vi "Zähler_konfigurieren_FGV.vi"(0 "Band/Station Index":T4, 1 "Modus":T3(ring), 3 "Konfiguration":T2, 4 "Zähler":enum16{"Zähler 1", "Zähler 2", "Zähler 3"}(ring)) -> (6 "Zählerkonfig.":T1(array[cluster]), 7 "Werte verändert":bool)   [LabVIEW 2013, in "cRIO_FPGA_COMMUNICATION.lvlib"]
uses:
  TYPES/TYPE Station Index.ctl
  cRIO_FPGA_COMMUNICATION.lvlib
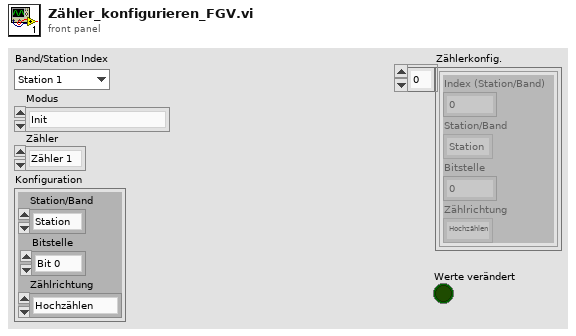
[diagram p1: front panel]
types:
  T1 = cluster{"Index (Station/Band)":u8, "Station/Band":enum16{"Station", "Band"}, "Bitstelle":u8, "Zählrichtung":enum16{"Hochzählen", "Runterzählen"}}[]
  T2 = typedef "TYPE Zählerkonfiguration.ctl" = cluster{"Station/Band":enum16{"Station", "Band"}, "Bitstelle":enum16{"Bit 0", "Bit 1", "Bit 2", "Bit 3", "Bit 4", "Bit 5", "Bit 6", "Bit 7"}, "Zählrichtung":enum16{"Hochzählen", "Runterzählen"}}
  T3 = enum16{"Init", "Zählerkonfig. setzen", "lese Zählerkonfig."}
  T4 = typedef "cRIO_FPGA_COMMUNICATION.lvlib/TYPE Station Index.ctl" = enum16{"Station 1", "Station 2", "Station 3", "Station 4", "Station 5", "Station 6", "Station 7", "Station 8", "Station 9", "Station 10", "Station 11", "Station 12", "Station 13", "Station 14", "Station 15", "Station 16", "Station 17", "Station 18", "Station 19", "Station 20"}
  T5 = cluster{"Index (Station/Band)":u8, "Station/Band":enum16{"Station", "Band"}, "Bitstelle":u8, "Zählrichtung":enum16{"Hochzählen", "Runterzählen"}}
  T6 = enum16{"Bit 0", "Bit 1", "Bit 2", "Bit 3", "Bit 4", "Bit 5", "Bit 6", "Bit 7"}
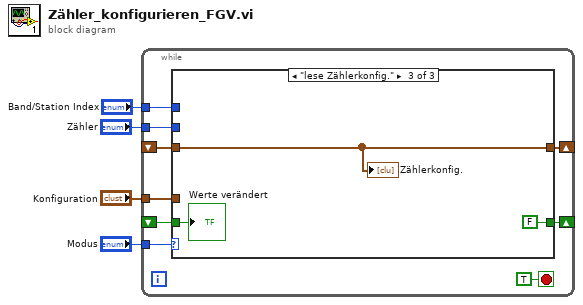
[diagram p0: block diagram]
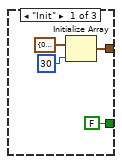
[diagram p2: hidden frame]
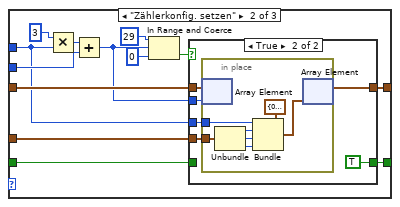
[diagram p3: hidden frame]
diagram:
  n1 = while {
    tunnel: "Modus" -> [w12]
    tunnel: "Konfiguration" -> [w11]
    tunnel: "Band/Station Index" -> [w10]
    tunnel: "Zähler" -> [w9]
    shift-right: [w7] -> _
    shift-left: _ -> [w8]
    shift-right: [w6] -> _
    shift-left: _ -> [w5]
    stop <- TRUE stop-if-true
    n2 = case shown="\"lese Zählerkonfig.\"" w12 {
      tunnel: w11 -> [_ w25 _]
      tunnel: w10 -> [_ w20 _]
      tunnel: w9 -> [_ w28 _]
      tunnel: [w16 w26 w48] -> w7
      tunnel: w8 -> [_ w27 w48]
      tunnel: [FALSE w19 FALSE] -> w6
      tunnel: w5 -> [_ w18 w46]
      frame "Init" {
        n3 = Initialize Array(T5 {"Index (Station/Band)"=0, "Station/Band"=enum."Station", "Bitstelle"=0, "Zählrichtung"=enum."Hochzählen"} ("Cluster"), 30 ("Dimension")) -> (w16:T1)
      }
      frame "Zählerkonfig. setzen" {
        n4 = Multiply(x=3, y=w20) -> (x*y=w30:i32)
        n5 = Add(x=w30, y=w28) -> (x+y=w21:i32)
        n6 = In Range and Coerce(upper limit=29 ("Obergrenze"), x=w21, lower limit=0 ("Untergrenze")) -> (In Range?=w22:bool)  [unwired: 1 out]
        n7 = case shown="True" w22 {
          tunnel: w27 -> [w32 w38]
          tunnel: [w32 w37] -> w26
          tunnel: w25 -> [_ w36]
          tunnel: w21 -> [_ w35]
          tunnel: w20 -> [_ w34]
          tunnel: [w31 TRUE] -> w19
          tunnel: w18 -> [w31 _]
          frame False {
          }
          frame True {
            n8 = in-place {
              in-place-border: w36 -> [w45]
              in-place-border: w34 -> [w40]
              n9 = in-place-array #1(w38, w35) -> ()  [unwired: 1 out]
              n10 = Unbundle(w45) -> ("Station/Band"=w41:enum16{"Station", "Band"}, "Bitstelle"=w42:T6, "Zählrichtung"=w43:enum16{"Hochzählen", "Runterzählen"})
              n11 = Bundle(cluster=T5 {"Index (Station/Band)"=0, "Station/Band"=enum."Station", "Bitstelle"=0, "Zählrichtung"=enum."Hochzählen"} ("Cluster"), "Index (Station/Band)"=w40, "Station/Band"=w41, "Bitstelle"=w42, "Zählrichtung"=w43) -> (w39:T5)
              n12 = in-place-array #1(w39) -> (w37:T1)  [unwired: 1 out]
            }
          }
        }
      }
      frame "lese Zählerkonfig." {
        "Zählerkonfig." <- w48
        "Werte verändert" <- w46
      }
    }
  }
